vi "ParseCommand_Parse_v4c.vi"(0 "Input":T3={"Temperature Map (full)"=[], "Temperature position"={"x"=0.0, "y"=0.0}, "Paths for files"=[], "Frame"=0.0, "Size"={"Height"=0.0, "Width"=0.0}, "Loop Size"=0.0, "Parsed command"="", "Binning"=1.0, "Dark pictures"=[]} {"Binning" min=1.0}, 1 "Temperature Assigned function":T4[](array[typedef]), 2 "1D Assigned function":T6[](array[typedef]), 3 "2D Assigned function":T5[](array[typedef]), 4 "Special Commands":T2[](array[typedef]), 5 "Picture areas":T1[](array[typedef]), 7 "Overexposure threshold":dbl) -> (6 "Output":dbl[][](graph), 8 "Overexposure?":bool)   [LabVIEW 2010]
uses:
  1DAssignedFunction.ctl
  Corrections.ctl
  2DAssignedFunction.ctl
  PictureAreaControl.ctl
  TemperatureAssignedFunction.ctl
  ParseInput.ctl
  SepcialCommands.ctl
  <vilib>/gmath/NI_Gmath.lvlib
  <vilib>/Analysis/NI_AALBase.lvlib
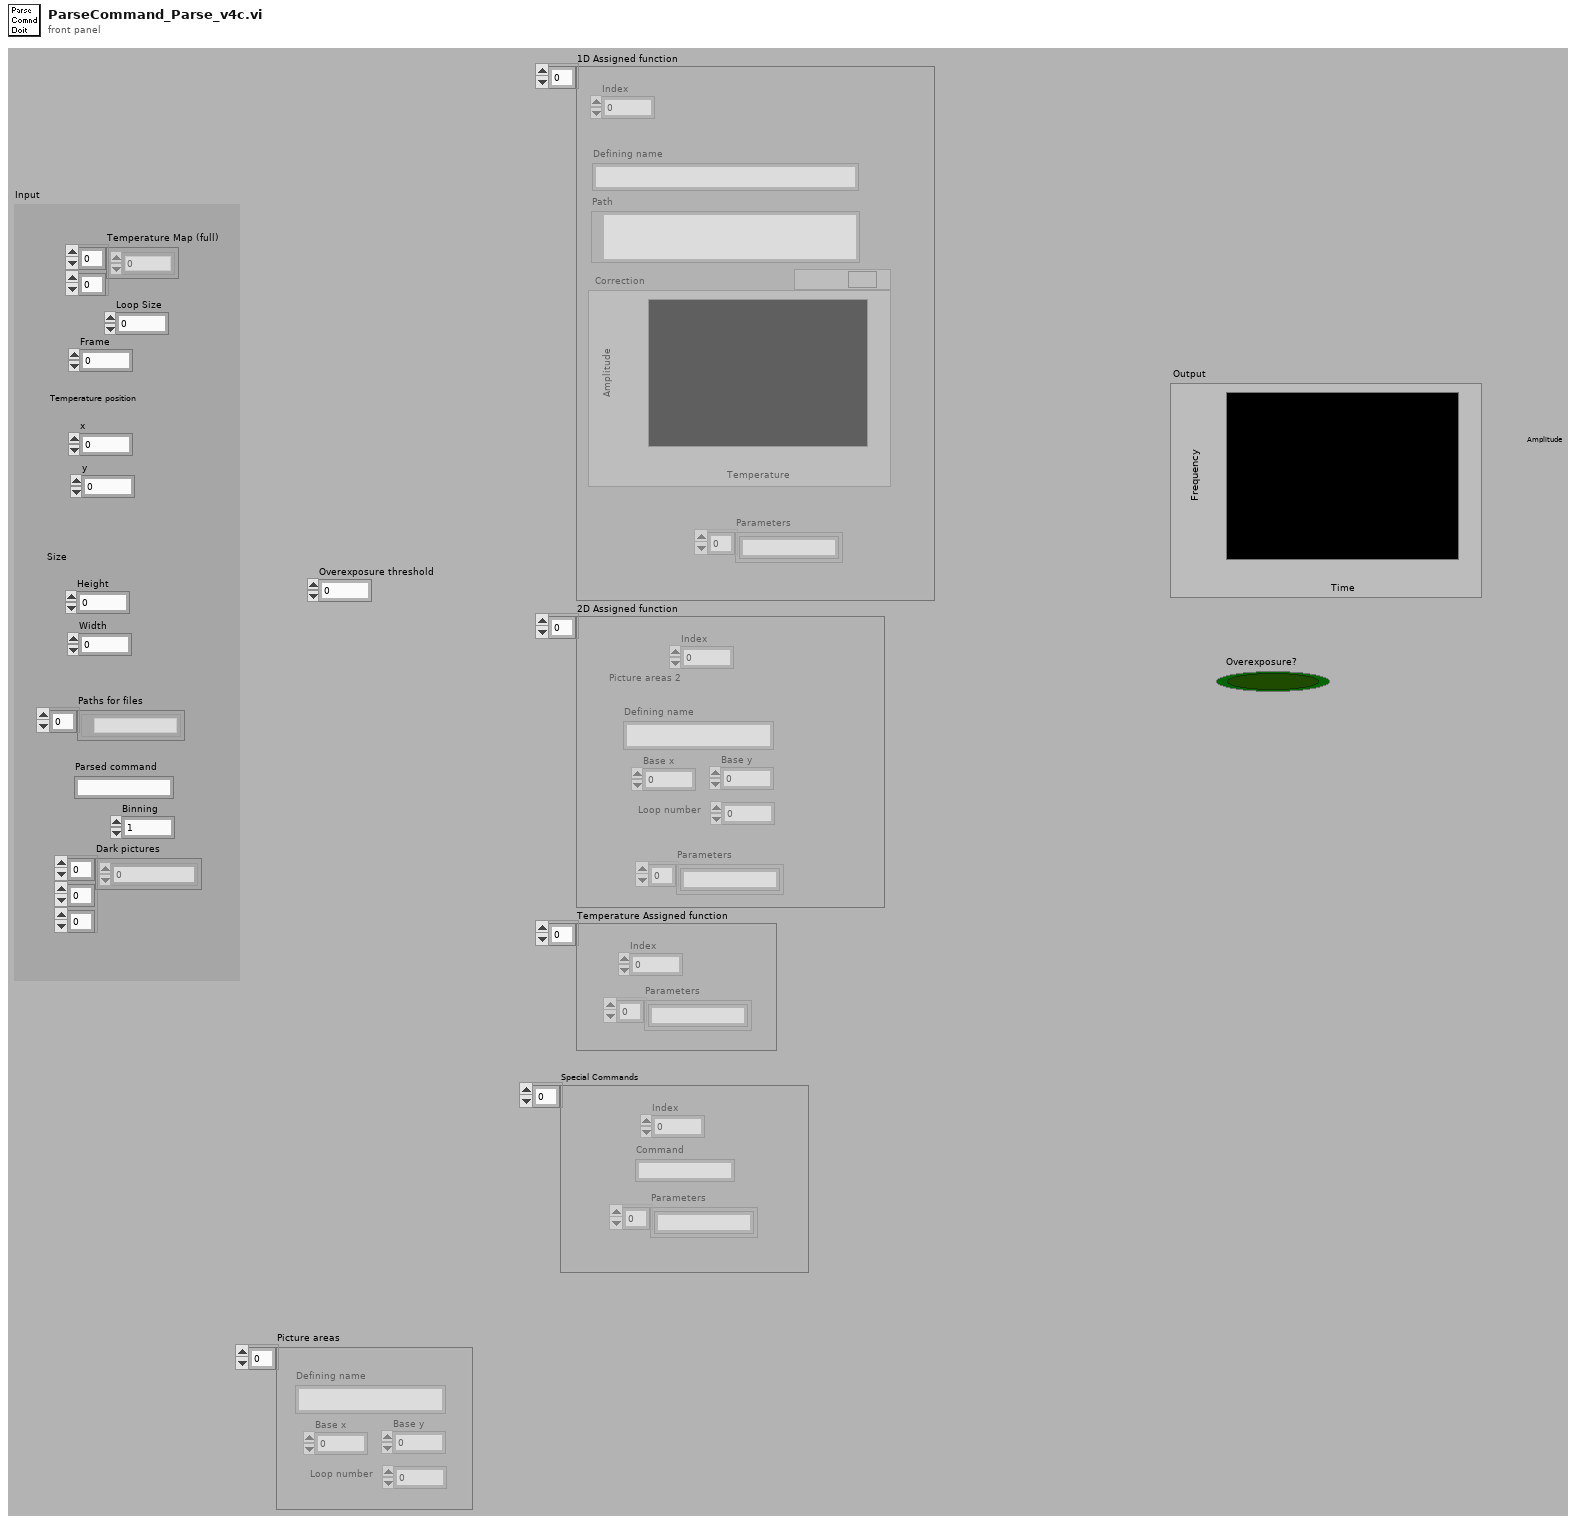
[diagram p1: front panel]
types:
  T1 = typedef "PictureAreaControl.ctl" = cluster{"Defining name":string, "Base x":dbl, "Base y":dbl, "Loop number":dbl}
  T2 = typedef "SepcialCommands.ctl" = cluster{"Index":dbl, "Command":string, "Parameters":string[]}
  T3 = typedef "ParseInput.ctl" = cluster{"Temperature Map (full)":dbl[][], "Temperature position":cluster{"x":dbl, "y":dbl}, "Paths for files":path[], "Frame":dbl, "Size":cluster{"Height":dbl, "Width":dbl}, "Loop Size":dbl, "Parsed command":string, "Binning":dbl, "Dark pictures":dbl[][][]}
  T4 = typedef "TemperatureAssignedFunction.ctl" = cluster{"Index":dbl, "Parameters":string[]}
  T5 = typedef "2DAssignedFunction.ctl" = cluster{"Index":dbl, "Picture areas 2":T1, "Parameters":string[]}
  T6 = typedef "1DAssignedFunction.ctl" = cluster{"Index":dbl, "Corrections":T7, "Parameters":string[]}
  T7 = typedef "Corrections.ctl" = cluster{"Path":path, "Defining name":string, "Correction":cluster{dbl, dbl}[]}
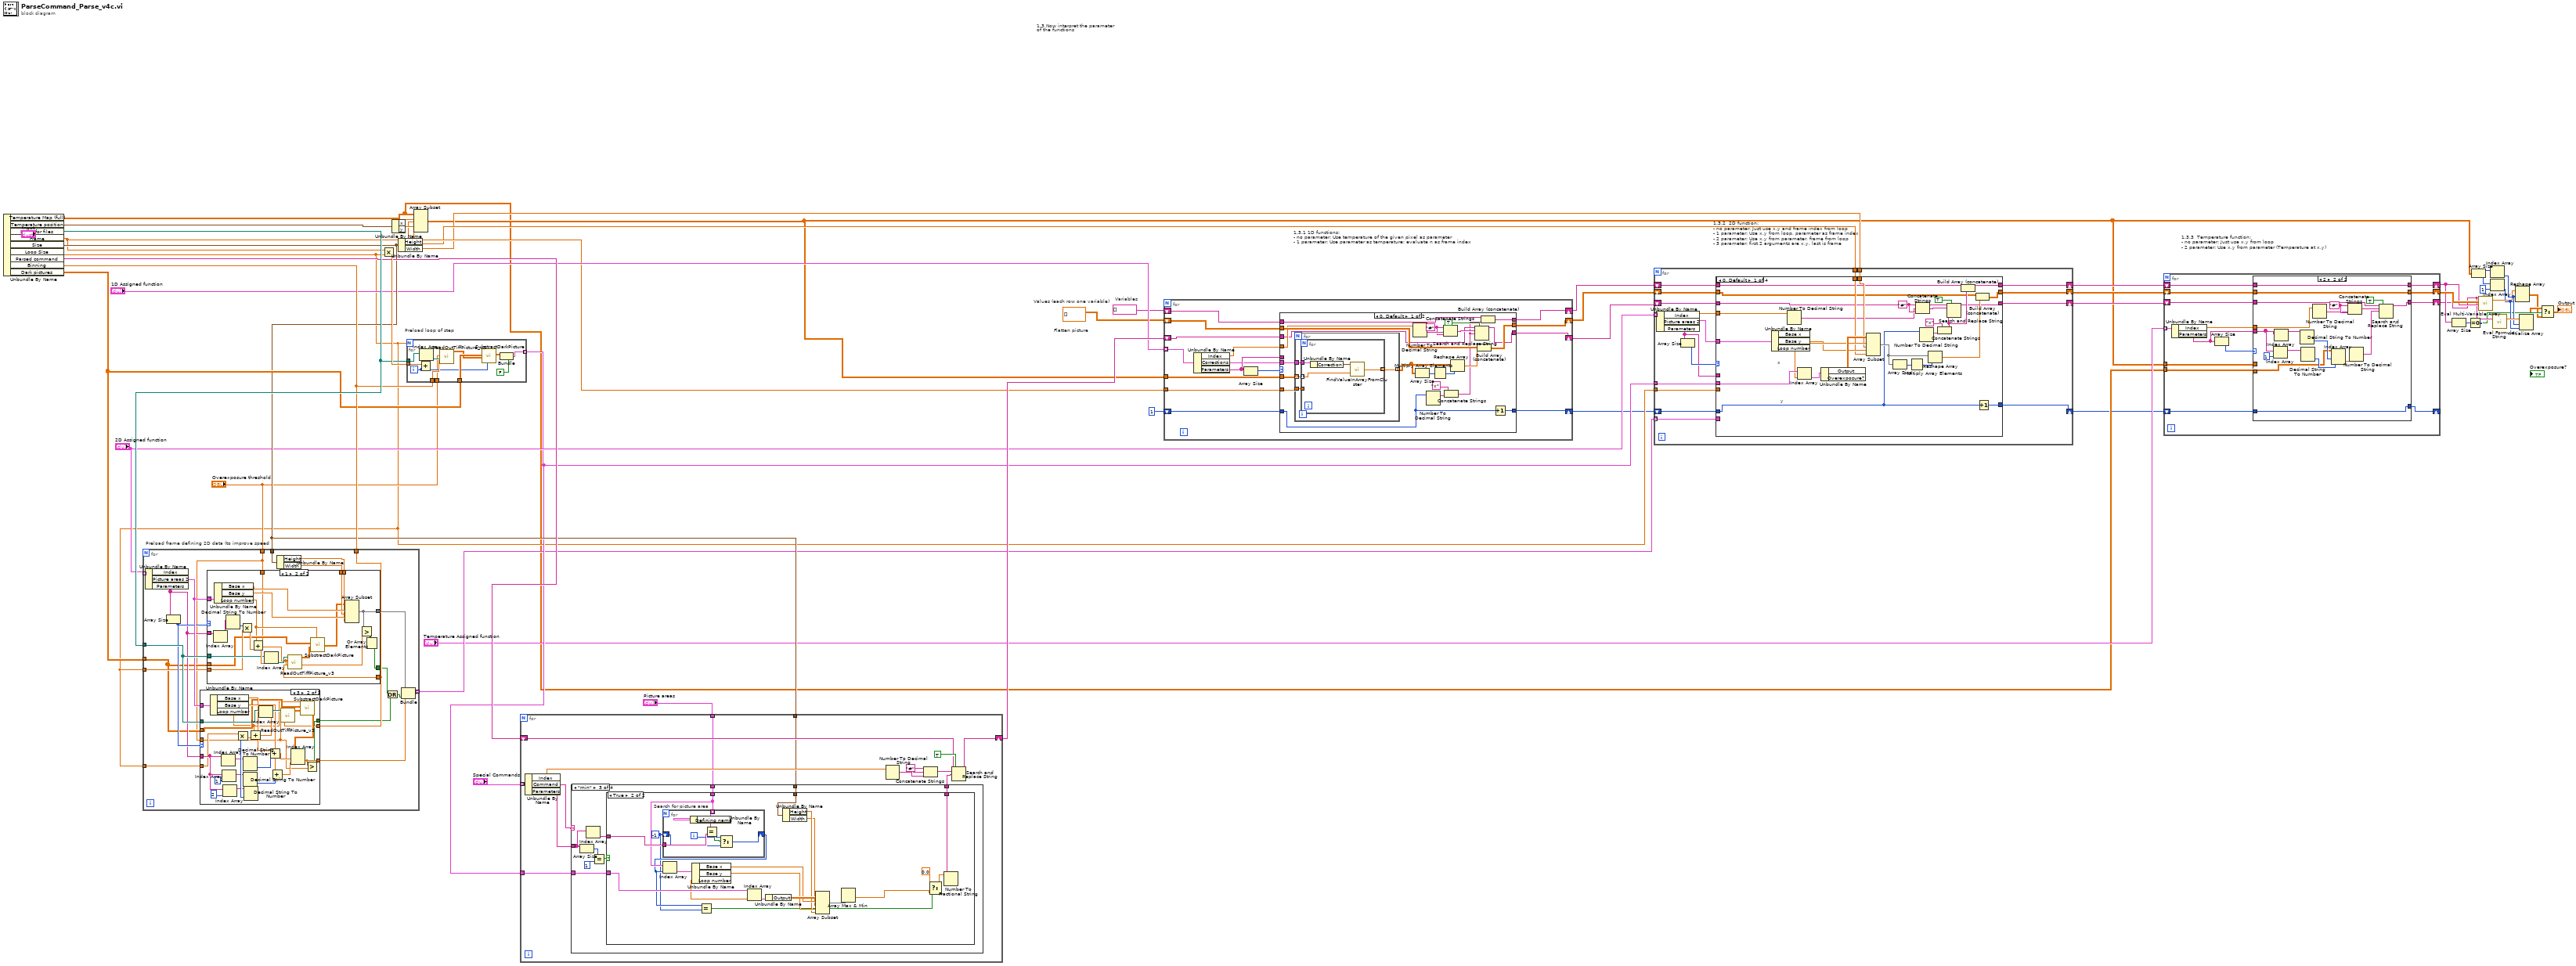
[diagram p0: block diagram]
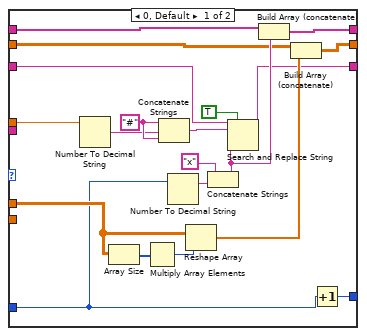
[diagram p2: hidden frame]
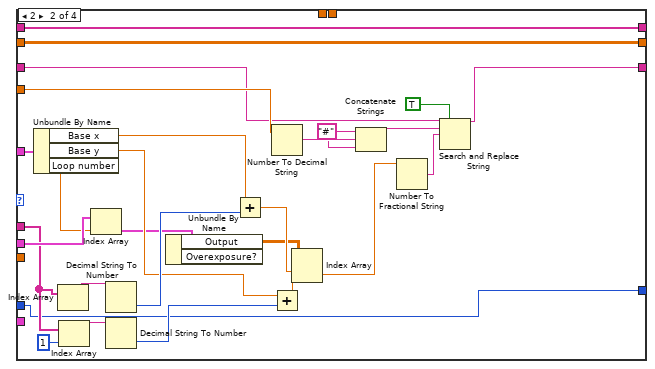
[diagram p3: hidden frame]
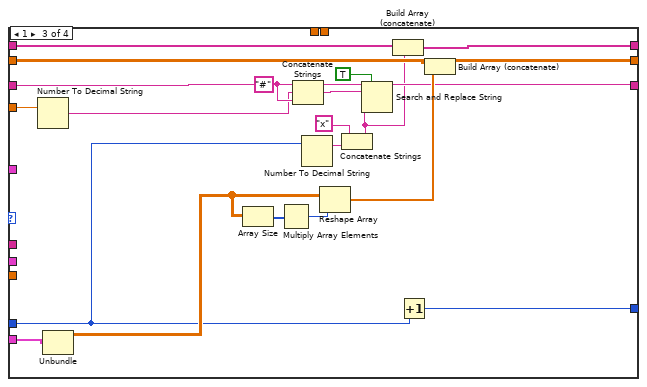
[diagram p4: hidden frame]
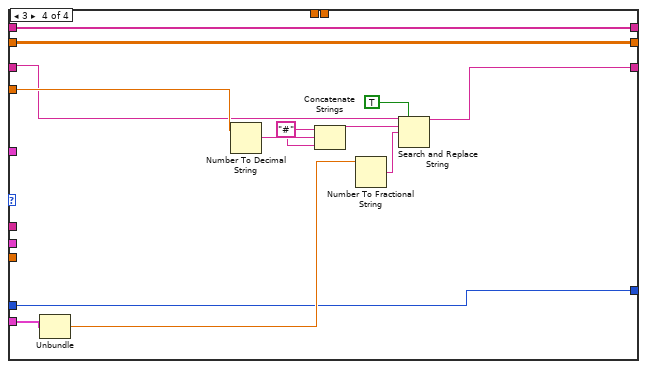
[diagram p5: hidden frame]
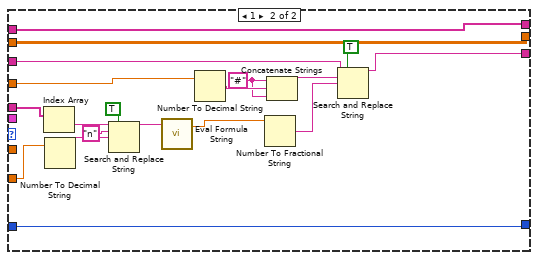
[diagram p6: hidden frame]
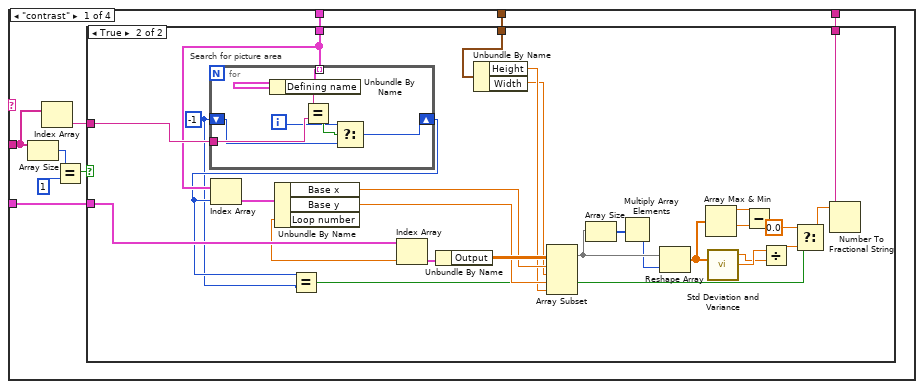
[diagram p7: hidden frame]
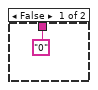
[diagram p8: hidden frame]
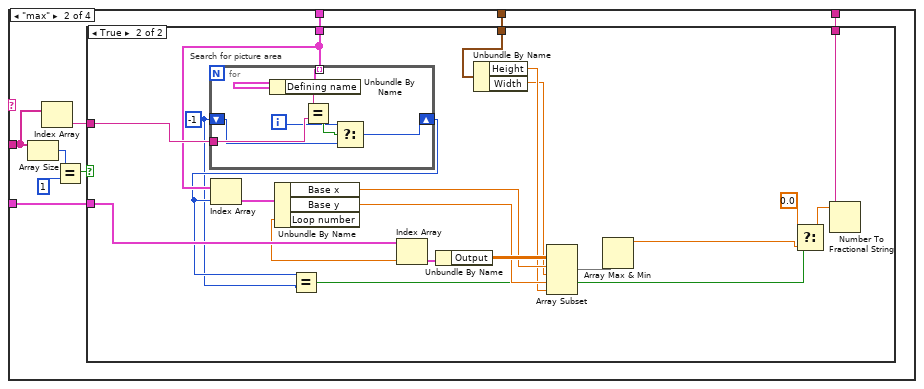
[diagram p9: hidden frame]
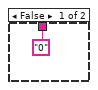
[diagram p10: hidden frame]
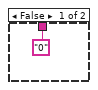
[diagram p11: hidden frame]
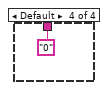
[diagram p12: hidden frame]
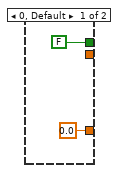
[diagram p13: hidden frame]
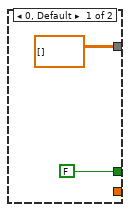
[diagram p14: hidden frame]
diagram:
  # "1.3.3  Temperature function:\n- no parameter: Just use x,y from loop\n- 2 parameter: Use x,y from parameter (Temperature at x,y)"
  # "1.3.2  2D function:\n- no parameter: Just use x,y and frame index from loop\n- 1 parameter: Use x,y from loop, parameter as frame index\n- 2 parameter: Use x,y from parameter, frame from loop\n- 3 parameter: first 2 arguments are x,y, last is frame"
  # "Values (each row one variable)"
  # "Flatten picture"
  # "Variables"
  # "1.3.1 1D functions:\n- no parameter: Use temperature of the given pixel as parameter\n- 1 parameter: Use parameter as temperature; evaluate n as frame index"
  # "Preload frame defining 2D data (to improve speed"
  # "Preload loop of step"
  # "1.3 Now interpret the parameter\nof the functions"
  n1 = Unbundle By Name("Input") -> ("Temperature Map (full)"=w14:dbl[][], "Temperature position"=w49:cluster{"x":dbl, "y":dbl}, "Paths for files"=w45:path[], "Frame"=w34:dbl, "Size"=w40:cluster{"Height":dbl, "Width":dbl}, "Loop Size"=w28:dbl, "Parsed command"=w42:string, "Binning"=w44:dbl, "Dark pictures"=w43:dbl[][][])
  n2 = for {
    tunnel: "2D Assigned function" -> [w69] mode=indexing
    tunnel: w45 -> [w68]
    tunnel: w40 -> [w62]
    tunnel: w28 -> [w64]
    tunnel: [w58] -> w27 mode=indexing
    tunnel: w28 -> [w57]
    tunnel: w44 -> [w56]
    tunnel: w43 -> [w55]
    tunnel: "Overexposure threshold" -> [w54]
    n3 = Unbundle By Name(w69) -> ("Picture areas 2"=w67:T1, "Parameters"=w65:string[])  [unwired: 1 out]
    n4 = Array Size(array=w65) -> (size(s)=w66:i32)
    n5 = case shown="3" w66 {
      tunnel: w68 -> [_ w93]
      tunnel: w67 -> [_ w92]
      tunnel: w65 -> [_ w91]
      tunnel: w64 -> [_ w90]
      tunnel: [0.0 w74] -> w63
      tunnel: w56 -> [_ w77]
      tunnel: w55 -> [_ w76]
      tunnel: w54 -> [_ w73]
      tunnel: [FALSE ("Overexposure?") w72] -> w52
      frame 0, Default {
      }
      frame 3 {
        n6 = Unbundle By Name(w92) -> ("Base x"=w84:dbl, "Base y"=w86:dbl, "Loop number"=w75:dbl)
        n7 = Index Array(array=w91) -> (element=w83:string)  [unwired: 1 in]
        n8 = Index Array(array=w91, index=1) -> (element=w82:string)
        n9 = Index Array(array=w91, index=2) -> (element=w81:string)
        n10 = Decimal String To Number(string=w83) -> (number=w85:i32)  [unwired: 2 in, 1 out]
        n11 = Decimal String To Number(string=w82) -> (number=w80:i32)  [unwired: 2 in, 1 out]
        n12 = Decimal String To Number(string=w81) -> (number=w96:i32)  [unwired: 2 in, 1 out]
        n13 = Multiply(x=w90, y=w96) -> (x*y=w95:dbl)
        n14 = Add(x=w75, y=w95) -> (x+y=w94:dbl)
        n15 = Index Array(array=w93, index=w94) -> (element=w89:path)
        n16 = Add(x=w84, y=w85) -> (x+y=w88:dbl)
        n17 = Add(x=w86, y=w80) -> (x+y=w87:dbl)
        n18 = call "ReadOutTiffPicture_v3.vi"("Binning size"=w77, "Overexposure threshold"=w73, "Path"=w89) -> ("Indicator"=w79:dbl[][])  [unwired: 1 in, 3 out]
        n19 = call "SubstractDarkPicture.vi"("Dark Pictures"=w76, "Input"=w79, "Loop index"=w75) -> ("Output"=w78:dbl[][])  [unwired: 2 in]
        n20 = Index Array(array=w78, index (row)=w88, index (col)=w87) -> (element=w74:dbl)
        n21 = Greater?(x=w74, y=w73) -> (0:w72:bool)
      }
    }
    n22 = Unbundle By Name(w62) -> ("Height"=w61:dbl, "Width"=w60:dbl)
    n23 = case shown="1" w66 {
      tunnel: w67 -> [_ w122]
      tunnel: w65 -> [_ w121]
      tunnel: w68 -> [_ w116]
      tunnel: w61 -> [_ w112]
      tunnel: w60 -> [_ w111]
      tunnel: [dbl[][] [] w104] -> w59
      tunnel: w57 -> [_ w110]
      tunnel: w56 -> [_ w109]
      tunnel: w55 -> [_ w106]
      tunnel: w54 -> [_ w103]
      tunnel: [FALSE ("Overexposure?") w101] -> w53
      frame 0, Default {
      }
      frame 1 {
        n24 = Index Array(array=w121) -> (element=w119:string)  [unwired: 1 in]
        n25 = Unbundle By Name(w122) -> ("Base x"=w114:dbl, "Base y"=w113:dbl, "Loop number"=w105:dbl)
        n26 = Decimal String To Number(string=w119) -> (number=w118:i32)  [unwired: 2 in, 1 out]
        n27 = Multiply(x=w118, y=w110) -> (x*y=w117:dbl)
        n28 = Add(x=w105, y=w117) -> (x+y=w120:dbl)
        n29 = Index Array(array=w116, index=w120) -> (element=w115:path)
        n30 = call "ReadOutTiffPicture_v3.vi"("Binning size"=w109, "Overexposure threshold"=w103, "Path"=w115) -> ("Indicator"=w108:dbl[][])  [unwired: 1 in, 3 out]
        n31 = call "SubstractDarkPicture.vi"("Dark Pictures"=w106, "Input"=w108, "Loop index"=w105) -> ("Output"=w107:dbl[][])  [unwired: 2 in]
        n32 = Array Subset(array=w107, index (row)=w114, length (row)=w111, index (col)=w113, length (col)=w112) -> (w104:dbl[][])
        n33 = Greater?(x=w104, y=w103) -> (0:w102:bool[][])
        n34 = Or Array Elements(Boolean array=w102) -> (logical OR=w101:bool)
      }
    }
    n35 = Or(x=w53, y=w52) -> (x .or. y?=w51:bool)
    n36 = Bundle(w59, w63, w51) -> (w58:cluster{dbl[][], dbl, bool})  [unwired: 1 in]
  }
  n37 = Multiply(x=w34, y=w28) -> (x*y=w46:dbl)
  n38 = Unbundle By Name(w49) -> ("x"=w48:dbl, "y"=w47:dbl)
  n39 = Unbundle By Name(w40) -> ("Height"=w21:dbl, "Width"=w20:dbl)
  n40 = for {
    N: w28 -> [_]
    tunnel: w45 -> [w133]
    tunnel: w46 -> [w132]
    tunnel: w44 -> [w130]
    tunnel: w43 -> [w129]
    tunnel: "Overexposure threshold" -> [w126]
    tunnel: [w124] -> w30 mode=indexing
    i -> [w128]
    n41 = Add(x=w132, y=w128) -> (x+y=w131:dbl)
    n42 = Index Array(array=w133, index=w131) -> (element=w134:path)
    n43 = call "ReadOutTiffPicture_v3.vi"("Binning size"=w130, "Overexposure threshold"=w126, "Path"=w134) -> ("Indicator"=w127:dbl[][])  [unwired: 1 in, 3 out]
    n44 = call "SubstractDarkPicture.vi"("Dark Pictures"=w129, "Input"=w127, "Loop index"=w128) -> ("Output"=w125:dbl[][])  [unwired: 2 in]
    n45 = Bundle("Output"=w125, "Overexposure?"=FALSE) -> (w124:cluster{"Output":dbl[][], "Overexposure?":bool})  [unwired: 1 in]
  }
  n46 = Array Subset(array=w14, index (row)=w48, length (row)=w20, index (col)=w47, length (col)=w21) -> (w15:dbl[][])
  n47 = for {
    tunnel: "Special Commands" -> [w148] mode=indexing
    shift-right: [w142] -> w36
    shift-left: w42 -> [w143]
    tunnel: "Picture areas" -> [w138]
    tunnel: w30 -> [w137]
    tunnel: w40 -> [w136]
    w147 = "#" ("string")
    n48 = Unbundle By Name(w148) -> ("Index"=w145:dbl, "Command"=w140:string, "Parameters"=w139:string[])
    n49 = case shown="\"min\"" w140 {
      tunnel: w139 -> [w153 w197 w234 _]
      tunnel: w138 -> [w154 w198 w235 _]
      tunnel: w137 -> [w151 w195 w232 _]
      tunnel: w136 -> [w150 w194 w231 _]
      tunnel: [w149 w193 w230 "0"] -> w135
      frame "contrast" {
        n50 = Array Size(array=w153) -> (size(s)=w157:i32)
        n51 = Index Array(array=w153) -> (element=w152:string)  [unwired: 1 in]
        n52 = Equal?(x=w157, y=1) -> (x = y?=w155:bool)
        n53 = case shown="True" w155 {
          tunnel: w154 -> [_ w184]
          tunnel: w152 -> [_ w185]
          tunnel: w151 -> [_ w182]
          tunnel: w150 -> [_ w179]
          tunnel: ["0" w170] -> w149
          frame False {
          }
          frame True {
            w161 = -1
            # "Search for picture area"
            n54 = for {
              tunnel: w184 -> [w192] mode=indexing
              shift-right: [w186] -> w162
              shift-left: w161 -> [w187]
              tunnel: w185 -> [w190]
              i -> [w188]
              n55 = Unbundle By Name(w192) -> ("Defining name"=w191:string)
              n56 = Equal?(x=w191, y=w190) -> (x = y?=w189:bool)
              n57 = Select(t=w188, s=w189, f=w187) -> (s? t:f=w186:i32)
            }
            n58 = Index Array(array=w184, index=w162) -> (element=w183:T1)
            n59 = Unbundle By Name(w183) -> ("Base x"=w177:dbl, "Base y"=w176:dbl, "Loop number"=w181:dbl)
            n60 = Equal?(x=w162, y=w161) -> (x = y?=w160:bool)
            n61 = Index Array(array=w182, index=w181) -> (element=w180:cluster{"Output":dbl[][], "Overexposure?":bool})
            n62 = Unbundle By Name(w180) -> ("Output"=w178:dbl[][])
            n63 = Unbundle By Name(w179) -> ("Height"=w175:dbl, "Width"=w174:dbl)
            n64 = Array Subset(array=w178, index (row)=w177, length (row)=w174, index (col)=w176, length (col)=w175) -> (w173:dbl[][])
            n65 = Array Size(array=w173) -> (size(s)=w172:i32[])
            n66 = Multiply Array Elements(1:w172) -> (0:w171:i32)
            n67 = Reshape Array(w173, w171) -> (w166:dbl[])
            n68 = Array Max & Min(array=w166) -> (max value=w165:dbl, min value=w164:dbl)  [unwired: 2 out]
            n69 = call <vilib>:"Std Deviation and Variance.vi"("X"=w166) -> ("mean"=w168:dbl, "standard deviation"=w169:dbl)  [unwired: 1 in, 1 out]
            n70 = Subtract(x=w165, y=w164) -> ()  [unwired: 1 out]
            n71 = Divide(x=w169, y=w168) -> (x/y=w167:dbl)
            n72 = Select(t=0.0, s=w160, f=w167) -> (s? t:f=w163:dbl)
            n73 = Number To Fractional String(number=w163) -> (F-format string=w170:string)  [unwired: 3 in]
          }
        }
      }
      frame "max" {
        n74 = Array Size(array=w197) -> (size(s)=w201:i32)
        n75 = Index Array(array=w197) -> (element=w196:string)  [unwired: 1 in]
        n76 = Equal?(x=w201, y=1) -> (x = y?=w199:bool)
        n77 = case shown="True" w199 {
          tunnel: w198 -> [_ w221]
          tunnel: w196 -> [_ w222]
          tunnel: w195 -> [_ w219]
          tunnel: w194 -> [_ w216]
          tunnel: ["0" w210] -> w193
          frame False {
          }
          frame True {
            w207 = -1
            # "Search for picture area"
            n78 = for {
              tunnel: w221 -> [w229] mode=indexing
              shift-right: [w223] -> w208
              shift-left: w207 -> [w224]
              tunnel: w222 -> [w227]
              i -> [w225]
              n79 = Unbundle By Name(w229) -> ("Defining name"=w228:string)
              n80 = Equal?(x=w228, y=w227) -> (x = y?=w226:bool)
              n81 = Select(t=w225, s=w226, f=w224) -> (s? t:f=w223:i32)
            }
            n82 = Index Array(array=w221, index=w208) -> (element=w220:T1)
            n83 = Unbundle By Name(w220) -> ("Base x"=w214:dbl, "Base y"=w213:dbl, "Loop number"=w218:dbl)
            n84 = Equal?(x=w208, y=w207) -> (x = y?=w206:bool)
            n85 = Index Array(array=w219, index=w218) -> (element=w217:cluster{"Output":dbl[][], "Overexposure?":bool})
            n86 = Unbundle By Name(w217) -> ("Output"=w215:dbl[][])
            n87 = Unbundle By Name(w216) -> ("Height"=w212:dbl, "Width"=w211:dbl)
            n88 = Array Subset(array=w215, index (row)=w214, length (row)=w211, index (col)=w213, length (col)=w212) -> (w204:dbl[][])
            n89 = Array Max & Min(array=w204) -> (max value=w203:dbl)  [unwired: 3 out]
            n90 = Select(t=0.0, s=w206, f=w203) -> (s? t:f=w209:dbl)
            n91 = Number To Fractional String(number=w209) -> (F-format string=w210:string)  [unwired: 3 in]
          }
        }
      }
      frame "min" {
        n92 = Array Size(array=w234) -> (size(s)=w238:i32)
        n93 = Index Array(array=w234) -> (element=w233:string)  [unwired: 1 in]
        n94 = Equal?(x=w238, y=1) -> (x = y?=w236:bool)
        n95 = case shown="True" w236 {
          tunnel: w235 -> [_ w258]
          tunnel: w233 -> [_ w259]
          tunnel: w232 -> [_ w256]
          tunnel: w231 -> [_ w253]
          tunnel: ["0" w247] -> w230
          frame False {
          }
          frame True {
            w244 = -1
            # "Search for picture area"
            n96 = for {
              tunnel: w258 -> [w266] mode=indexing
              shift-right: [w260] -> w245
              shift-left: w244 -> [w261]
              tunnel: w259 -> [w264]
              i -> [w262]
              n97 = Unbundle By Name(w266) -> ("Defining name"=w265:string)
              n98 = Equal?(x=w265, y=w264) -> (x = y?=w263:bool)
              n99 = Select(t=w262, s=w263, f=w261) -> (s? t:f=w260:i32)
            }
            n100 = Index Array(array=w258, index=w245) -> (element=w257:T1)
            n101 = Unbundle By Name(w257) -> ("Base x"=w251:dbl, "Base y"=w250:dbl, "Loop number"=w255:dbl)
            n102 = Equal?(x=w245, y=w244) -> (x = y?=w243:bool)
            n103 = Index Array(array=w256, index=w255) -> (element=w254:cluster{"Output":dbl[][], "Overexposure?":bool})
            n104 = Unbundle By Name(w254) -> ("Output"=w252:dbl[][])
            n105 = Unbundle By Name(w253) -> ("Height"=w249:dbl, "Width"=w248:dbl)
            n106 = Array Subset(array=w252, index (row)=w251, length (row)=w248, index (col)=w250, length (col)=w249) -> (w241:dbl[][])
            n107 = Array Max & Min(array=w241) -> (min value=w240:dbl)  [unwired: 3 out]
            n108 = Select(t=0.0, s=w243, f=w240) -> (s? t:f=w246:dbl)
            n109 = Number To Fractional String(number=w246) -> (F-format string=w247:string)  [unwired: 3 in]
          }
        }
      }
      frame Default {
      }
    }
    n110 = Number To Decimal String(number=w145) -> (decimal integer string=w146:string)  [unwired: 1 in]
    n111 = Concatenate Strings(w147, w146, w147) -> (w141:string)
    n112 = Search and Replace String(replace all?=TRUE ("replace all? (F)"), input string=w143, search string=w141, replace string=w135) -> (result string=w142:string)  [unwired: 4 in, 3 out]
  }
  n113 = for {
    tunnel: "1D Assigned function" -> [w280] mode=indexing
    tunnel: w34 -> [w282]
    tunnel: w15 -> [w281]
    shift-right: [w272] -> w26
    shift-left: w36 -> [w276]
    shift-right: [w271] -> w25
    shift-left: string[] [] ("appended array") -> [w274]
    shift-right: [w270] -> w24
    shift-left: dbl[][] [] ("subarray") -> [w273]
    shift-right: [w268] -> w22
    shift-left: 1 -> [w269]
    n114 = Unbundle By Name(w280) -> ("Index"=w275:dbl, "Corrections"=w277:T7, "Parameters"=w278:string[])
    n115 = Array Size(array=w278) -> (size(s)=w279:i32)
    n116 = case shown="0, Default" w279 {
      tunnel: w282 -> [w305 w332]
      tunnel: w281 -> [w304 _]
      tunnel: w278 -> [_ w331]
      tunnel: w277 -> [w303 _]
      tunnel: w276 -> [w285 w319]
      tunnel: w275 -> [w292 w320]
      tunnel: [w284 w318] -> w272
      tunnel: w274 -> [w300 w316]
      tunnel: w273 -> [w295 w315]
      tunnel: [w296 w316] -> w271
      tunnel: [w293 w315] -> w270
      tunnel: w269 -> [w288 w314]
      tunnel: [w290 w314] -> w268
      frame 0, Default {
        w301 = "#" ("string")
        n117 = for {
          tunnel: w305 -> [w309]
          tunnel: w304 -> [w308] mode=indexing
          tunnel: w303 -> [w307]
          tunnel: [w306] -> w299 mode=indexing
          n118 = for {
            tunnel: w308 -> [w311] mode=indexing
            tunnel: w309 -> [_]
            tunnel: w307 -> [w312]
            tunnel: [w310] -> w306 mode=indexing
            n119 = Unbundle By Name(w312) -> ("Correction"=w313:cluster{dbl, dbl}[])
            n120 = call "FindValueInArrayFromCluster.vi"("Value"=w311, "Correction"=w313) -> ("Output"=w310:dbl)
          }
        }
        n121 = Number To Decimal String(number=w292) -> (decimal integer string=w302:string)  [unwired: 1 in]
        n122 = Array Size(array=w299) -> (size(s)=w298:i32[])
        n123 = Number To Decimal String(number=w288) -> (decimal integer string=w287:string)  [unwired: 1 in]
        n124 = Multiply Array Elements(1:w298) -> (0:w297:i32)
        n125 = Concatenate Strings(w301, w302, w301) -> (w291:string)
        n126 = Concatenate Strings("x" ("string"), w287) -> (w283:string)
        n127 = Reshape Array(w299, w297) -> (w294:dbl[])
        n128 = Search and Replace String(replace all?=TRUE ("replace all? (F)"), input string=w285, search string=w291, replace string=w283) -> (result string=w284:string)  [unwired: 4 in, 3 out]
        n129 = Build Array (concatenate)(w295, w294) -> (w293:dbl[][])
        n130 = Build Array (concatenate)(w300, w283) -> (w296:string[])
        n131 = Increment(x=w288) -> (x+1=w290:i32)
      }
      frame 1 {
        w324 = "#" ("string")
        n132 = Index Array(array=w331) -> (element=w328:string)  [unwired: 1 in]
        n133 = Number To Decimal String(number=w332) -> (decimal integer string=w327:string)  [unwired: 1 in]
        n134 = Search and Replace String(replace all?=TRUE ("replace all? (F)"), input string=w328, search string="n", replace string=w327) -> (result string=w326:string)  [unwired: 4 in, 3 out]
        n135 = call <vilib>:"Eval Formula String.vi"("formula"=w326) -> ("y value"=w321:dbl)  [unwired: 1 in, 1 out]
        n136 = Number To Decimal String(number=w320) -> (decimal integer string=w325:string)  [unwired: 1 in]
        n137 = Number To Fractional String(number=w321) -> (F-format string=w322:string)  [unwired: 3 in]
        n138 = Concatenate Strings(w324, w325, w324) -> (w323:string)
        n139 = Search and Replace String(replace all?=TRUE ("replace all? (F)"), input string=w319, search string=w323, replace string=w322) -> (result string=w318:string)  [unwired: 4 in, 3 out]
      }
    }
  }
  n140 = for {
    shift-right: [w337] -> w19
    shift-left: w26 -> [w343]
    tunnel: "2D Assigned function" -> [w350] mode=indexing
    tunnel: w30 -> [w348]
    tunnel: w28 -> [w346]
    tunnel: w27 -> [w344] mode=indexing
    shift-right: [w340] -> w18
    shift-left: w25 -> [w341]
    shift-right: [w339] -> w17
    shift-left: w24 -> [w338]
    shift-right: [w335] -> w11
    shift-left: w22 -> [w336]
    tunnel: w21 -> [w334]
    tunnel: w20 -> [w333]
    n141 = Unbundle By Name(w350) -> ("Index"=w342:dbl, "Picture areas 2"=w349:T1, "Parameters"=w345:string[])
    n142 = Array Size(array=w345) -> (size(s)=w347:i32)
    n143 = case shown="0, Default" w347 {
      tunnel: w349 -> [w379 w406 _ _]
      tunnel: w348 -> [w378 w405 _ _]
      tunnel: w346 -> [_ _ _ _]
      tunnel: w345 -> [_ w403 _ _]
      tunnel: w344 -> [_ _ w427 w440]
      tunnel: w343 -> [w358 w383 w415 w433]
      tunnel: [w355 w382 w411 w432] -> w337
      tunnel: w342 -> [w357 w384 w417 w434]
      tunnel: w341 -> [w354 w391 w410 w430]
      tunnel: [w353 w391 w408 w430] -> w340
      tunnel: [w352 w390 w407 w429] -> w339
      tunnel: w338 -> [w351 w390 w422 w429]
      tunnel: w336 -> [w359 w380 w412 w428]
      tunnel: [w375 w380 w426 w428] -> w335
      tunnel: w334 -> [w371 _ _ _]
      tunnel: w333 -> [w370 _ _ _]
      frame 0, Default {
        w364 = "#" ("string")
        # "y"
        # "x"
        n144 = Unbundle By Name(w379) -> ("Base x"=w373:dbl, "Base y"=w372:dbl, "Loop number"=w377:dbl)
        n145 = Number To Decimal String(number=w357) -> (decimal integer string=w356:string)  [unwired: 1 in]
        n146 = Index Array(array=w378, index=w377) -> (element=w376:cluster{"Output":dbl[][], "Overexposure?":bool})
        n147 = Unbundle By Name(w376) -> ("Output"=w374:dbl[][])  [unwired: 1 out]
        n148 = Array Subset(array=w374, index (row)=w373, length (row)=w370, index (col)=w372, length (col)=w371) -> (w360:dbl[][])
        n149 = Array Size(array=w360) -> (size(s)=w368:i32[])
        n150 = Multiply Array Elements(1:w368) -> (0:w369:i32)
        n151 = Concatenate Strings(w364, w356, w364) -> (w366:string)
        n152 = Number To Decimal String(number=w359) -> (decimal integer string=w363:string)  [unwired: 1 in]
        n153 = Reshape Array(w360, w369) -> (w367:dbl[])
        n154 = Concatenate Strings("x" ("string"), w363) -> (w361:string)
        n155 = Search and Replace String(replace all?=TRUE ("replace all? (F)"), input string=w358, search string=w366, replace string=w361) -> (result string=w355:string)  [unwired: 4 in, 3 out]
        n156 = Build Array (concatenate)(w354, w361) -> (w353:string[])
        n157 = Build Array (concatenate)(w351, w367) -> (w352:dbl[][])
        n158 = Increment(x=w359) -> (x+1=w375:i32)
      }
      frame 2 {
        w385 = "#" ("string")
        n159 = Unbundle By Name(w406) -> ("Base x"=w399:dbl, "Base y"=w396:dbl, "Loop number"=w404:dbl)
        n160 = Index Array(array=w403) -> (element=w401:string)  [unwired: 1 in]
        n161 = Index Array(array=w403, index=1) -> (element=w400:string)
        n162 = Index Array(array=w405, index=w404) -> (element=w393:cluster{"Output":dbl[][], "Overexposure?":bool})
        n163 = Decimal String To Number(string=w401) -> (number=w398:i32)  [unwired: 2 in, 1 out]
        n164 = Decimal String To Number(string=w400) -> (number=w395:i32)  [unwired: 2 in, 1 out]
        n165 = Unbundle By Name(w393) -> ("Output"=w392:dbl[][])  [unwired: 1 out]
        n166 = Add(x=w399, y=w398) -> (x+y=w397:dbl)
        n167 = Number To Decimal String(number=w384) -> (decimal integer string=w387:string)  [unwired: 1 in]
        n168 = Add(x=w396, y=w395) -> (x+y=w394:dbl)
        n169 = Index Array(array=w392, index (row)=w397, index (col)=w394) -> (element=w381:dbl)
        n170 = Concatenate Strings(w385, w387, w385) -> (w386:string)
        n171 = Number To Fractional String(number=w381) -> (F-format string=w388:string)  [unwired: 3 in]
        n172 = Search and Replace String(replace all?=TRUE ("replace all? (F)"), input string=w383, search string=w386, replace string=w388) -> (result string=w382:string)  [unwired: 4 in, 3 out]
      }
      frame 1 {
        w418 = "#" ("string")
        n173 = Number To Decimal String(number=w417) -> (decimal integer string=w416:string)  [unwired: 1 in]
        n174 = Unbundle(w427) -> (w423:dbl[][])  [unwired: 2 out]
        n175 = Array Size(array=w423) -> (size(s)=w424:i32[])
        n176 = Multiply Array Elements(1:w424) -> (0:w425:i32)
        n177 = Concatenate Strings(w418, w416, w418) -> (w420:string)
        n178 = Number To Decimal String(number=w412) -> (decimal integer string=w414:string)  [unwired: 1 in]
        n179 = Reshape Array(w423, w425) -> (w421:dbl[])
        n180 = Concatenate Strings("x" ("string"), w414) -> (w409:string)
        n181 = Search and Replace String(replace all?=TRUE ("replace all? (F)"), input string=w415, search string=w420, replace string=w409) -> (result string=w411:string)  [unwired: 4 in, 3 out]
        n182 = Build Array (concatenate)(w410, w409) -> (w408:string[])
        n183 = Increment(x=w412) -> (x+1=w426:i32)
        n184 = Build Array (concatenate)(w422, w421) -> (w407:dbl[][])
      }
      frame 3 {
        w435 = "#" ("string")
        n185 = Unbundle(w440) -> (w431:dbl)  [unwired: 2 out]
        n186 = Number To Decimal String(number=w434) -> (decimal integer string=w437:string)  [unwired: 1 in]
        n187 = Concatenate Strings(w435, w437, w435) -> (w436:string)
        n188 = Number To Fractional String(number=w431) -> (F-format string=w438:string)  [unwired: 3 in]
        n189 = Search and Replace String(replace all?=TRUE ("replace all? (F)"), input string=w433, search string=w436, replace string=w438) -> (result string=w432:string)  [unwired: 4 in, 3 out]
      }
    }
  }
  n190 = for {
    tunnel: "Temperature Assigned function" -> [w454] mode=indexing
    shift-right: [w441] -> w8
    shift-left: w19 -> [w449]
    tunnel: w15 -> [w452]
    tunnel: w14 -> [w450]
    shift-right: [w446] -> w10
    shift-left: w18 -> [w445]
    shift-right: [w448] -> w13
    shift-left: w17 -> [w447]
    shift-right: [w443] -> _
    shift-left: w11 -> [w444]
    n191 = Unbundle By Name(w454) -> ("Index"=w442:dbl, "Parameters"=w451:string[])
    n192 = Array Size(array=w451) -> (size(s)=w453:i32)
    n193 = case shown="2" w453 {
      tunnel: w452 -> [w465 _]
      tunnel: w451 -> [_ w492]
      tunnel: w450 -> [_ w487]
      tunnel: w449 -> [w456 w479]
      tunnel: [w455 w477] -> w441
      tunnel: [w459 w484] -> w448
      tunnel: w447 -> [w460 w484]
      tunnel: [w461 w485] -> w446
      tunnel: w445 -> [w462 w485]
      tunnel: w444 -> [w463 w486]
      tunnel: [w464 w486] -> w443
      tunnel: w442 -> [w458 w478]
      frame 0, Default {
        w471 = "#" ("string")
        n194 = Number To Decimal String(number=w458) -> (decimal integer string=w457:string)  [unwired: 1 in]
        n195 = Array Size(array=w465) -> (size(s)=w467:i32[])
        n196 = Multiply Array Elements(1:w467) -> (0:w466:i32)
        n197 = Concatenate Strings(w471, w457, w471) -> (w469:string)
        n198 = Number To Decimal String(number=w463) -> (decimal integer string=w472:string)  [unwired: 1 in]
        n199 = Reshape Array(w465, w466) -> (w468:dbl[])
        n200 = Concatenate Strings("x" ("string"), w472) -> (w474:string)
        n201 = Search and Replace String(replace all?=TRUE ("replace all? (F)"), input string=w456, search string=w469, replace string=w474) -> (result string=w455:string)  [unwired: 4 in, 3 out]
        n202 = Build Array (concatenate)(w462, w474) -> (w461:string[])
        n203 = Build Array (concatenate)(w460, w468) -> (w459:dbl[][])
        n204 = Increment(x=w463) -> (x+1=w464:i32)
      }
      frame 2 {
        w483 = "#" ("string")
        n205 = Index Array(array=w492, index=1) -> (element=w490:string)
        n206 = Index Array(array=w492) -> (element=w491:string)  [unwired: 1 in]
        n207 = Decimal String To Number(string=w491) -> (number=w489:i32)  [unwired: 2 in, 1 out]
        n208 = Decimal String To Number(string=w490) -> (number=w488:i32)  [unwired: 2 in, 1 out]
        n209 = Number To Decimal String(number=w478) -> (decimal integer string=w480:string)  [unwired: 1 in]
        n210 = Index Array(array=w487, index (row)=w489, index (col)=w488) -> (element=w476:dbl)
        n211 = Concatenate Strings(w483, w480, w483) -> (w481:string)
        n212 = Number To Decimal String(number=w476) -> (decimal integer string=w475:string)  [unwired: 1 in]
        n213 = Search and Replace String(replace all?=TRUE ("replace all? (F)"), input string=w479, search string=w481, replace string=w475) -> (result string=w477:string)  [unwired: 4 in, 3 out]
      }
    }
  }
  n214 = Array Size(array=w10) -> (size(s)=w9:i32)
  n215 = Equal To 0?(x=w9) -> (x = 0?=w4:bool)
  n216 = Array Size(array=w15) -> (size(s)=w37:i32[])
  n217 = call <vilib>:"Eval Multi-Variable Array.vi"("Variables"=w10, "X Values"=w13, "formula"=w8) -> ("Y Values"=w12:dbl[])  [unwired: 1 in, 1 out]
  n218 = Index Array(array=w37) -> (element=w6:i32)  [unwired: 1 in]
  n219 = Index Array(array=w37, index=1) -> (element=w5:i32)
  n220 = call <vilib>:"Eval Formula String.vi"("formula"=w8) -> ("y value"=w7:dbl)  [unwired: 1 in, 1 out]
  n221 = Reshape Array(w12, w6, w5) -> (w2:dbl[][])
  n222 = Initialize Array(w7, w6, w5) -> (w3:dbl[][])
  n223 = Select(t=w3, s=w4, f=w2) -> (s? t:f=→"Output":dbl[][])
